vi "GetLastError.vi"(4 "error in (no error)":errorcluster) -> (0 "error out":errorcluster, 3 "CODE":i32)   [LabVIEW 2011]
uses:
  kernel32.dll
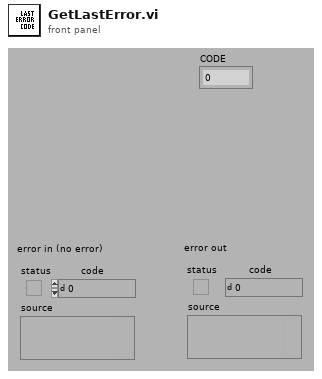
[diagram p1: front panel]
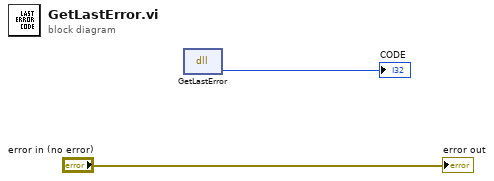
[diagram p0: block diagram]
diagram:
  n1 = dll-call lib="kernel32.dll" fn="GetLastError"() -> ("CODE"=→"CODE":i32)  [unwired: 3 in, 2 out]
  "error out" <- "error in (no error)"
